vi "Open Label.vi"(8 "error in (no error)":errorcluster) -> (0 "error out":errorcluster, 1 "ME79 Fail":refnum<k7>, 2 "ME79 Pass":refnum<k7>, 3 "reference out":refnum<k7>)   [LabVIEW 2018]
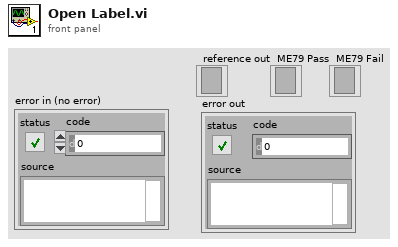
[diagram p1: front panel]
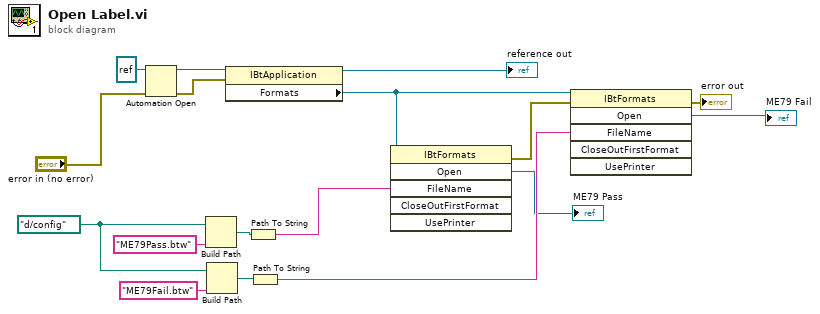
[diagram p0: block diagram]
diagram:
  w8 = path "d:/config" ("base path")
  n1 = Automation Open(error in (no error)="error in (no error)", Automation Refnum=refnum<k7> refnum ("BarTender.IBtApplication")) -> (Automation Refnum=w15:refnum<k7>, error out=w14:errorcluster)  [unwired: 2 in]
  n2 = Build Path(base path=w8, name or relative path="ME79Pass.btw") -> (appended path=w11:path)
  n3 = Build Path(base path=w8, name or relative path="ME79Fail.btw") -> (appended path=w4:path)
  n4 = property class="IBtApplication"(reference=w15, error in=w14) -> (reference out=→"reference out":refnum<k7>, "Formats"=w7:refnum<k7>)  [unwired: 1 out]
  n5 = Path To String(path=w11) -> (string=w10:string)
  n6 = Path To String(path=w4) -> (string=w3:string)
  n7 = invoke class="IBtFormats" method="Open"(reference=w7, "FileName"=w10) -> (error out=w6:errorcluster, "Open"=→"ME79 Pass":refnum<k7>)  [unwired: 4 in, 4 out]
  n8 = invoke class="IBtFormats" method="Open"(reference=w7, error in=w6, "FileName"=w3) -> (error out=→"error out":errorcluster, "Open"=→"ME79 Fail":refnum<k7>)  [unwired: 3 in, 4 out]
